vi "Write Samples per write.vi"(8 "error in (no error)":errorcluster, 10 "Samples per write":i32=-1, 11 "Pulse Driver in":refnum<class "Pulse Driver.lvclass">) -> (0 "error out":errorcluster, 3 "Pulse Driver out":refnum<class "Pulse Driver.lvclass">)   [LabVIEW 2020, in "Pulse Driver.lvclass"]
uses:
  Pulse Driver.lvclass
  Pulse Driver.lvclass/Pulse Driver.ctl
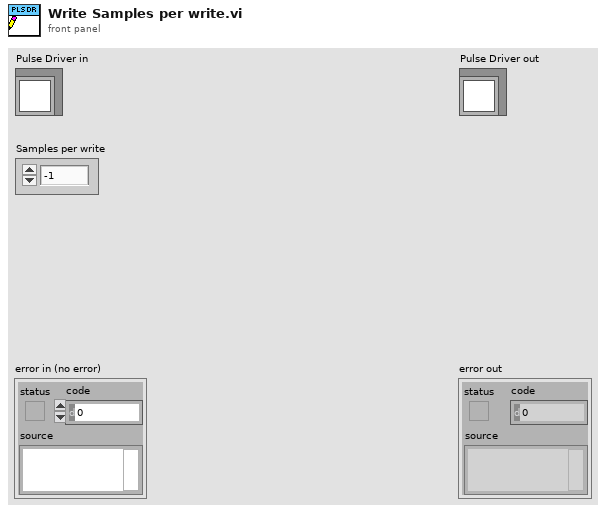
[diagram p1: front panel]
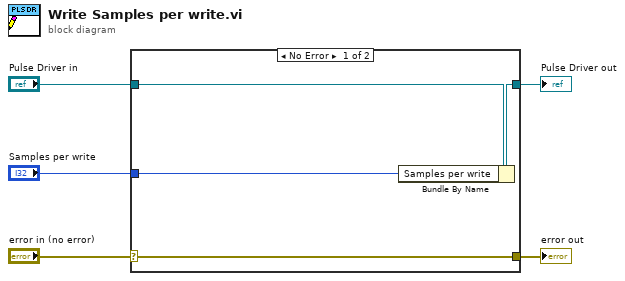
[diagram p0: block diagram]
diagram:
  n1 = case shown="No Error" "error in (no error)" {
    selector: "error in (no error)" -> [w9 w10]
    tunnel: [w9 w10] -> w4
    tunnel: [w7 w11] -> w2
    tunnel: "Pulse Driver in" -> [w8 w11]
    tunnel: "Samples per write" -> [w6 _]
    frame No Error {
      n2 = Bundle By Name(cluster=w8, "Samples per write"=w6) -> (w7:refnum<class "Pulse Driver.lvclass">)
    }
    frame Error {
    }
  }
  "error out" <- w4
  "Pulse Driver out" <- w2
